vi "update unit ID.vi"(8 "error in (no error)":errorcluster, 11 "Modbus Module runtime in":refnum<class "Modbus Module runtime.lvclass">) -> (0 "error out":errorcluster, 3 "Modbus Module runtime out":refnum<class "Modbus Module runtime.lvclass">)   [LabVIEW 2015, in "Modbus Module runtime.lvclass"]
uses:
  Modbus Module runtime.lvclass
  Modbus Module runtime.lvclass/Modbus Module runtime.ctl
  <vilib>/NI/Modbus Library/API/Modbus API.lvclass/Modbus API.ctl
  <vilib>/NI/Modbus Library/Transmission Data Unit/Transmission Data Unit.lvclass/Transmission Data Unit.ctl
  <vilib>/NI/Modbus Library/Transmission Data Unit/Transmission Data Unit.lvclass
  <vilib>/NI/Modbus Library/API/Modbus API.lvclass
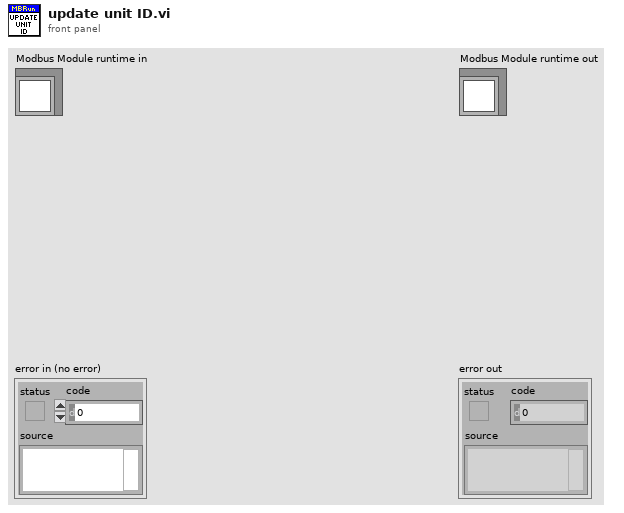
[diagram p1: front panel]
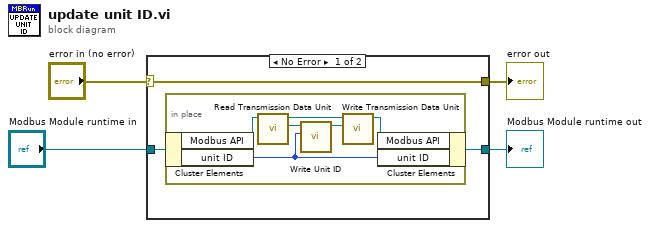
[diagram p0: block diagram]
diagram:
  n1 = case shown="No Error" "error in (no error)" {
    selector: "error in (no error)" -> [w7 w15]
    tunnel: [w7 w15] -> w3
    tunnel: [w5 w14] -> w1
    tunnel: "Modbus Module runtime in" -> [w6 w14]
    frame No Error {
      n2 = in-place {
        n3 = in-place-cluster #1(w6) -> ("Modbus API"=w13:refnum<class "Modbus API.lvclass">, "unit ID"=w8:u8)
        n4 = call <vilib>:"Read Transmission Data Unit.vi"("Modbus instance in"=w13) -> ("transmission data unit"=w12:refnum<class "Transmission Data Unit.lvclass">, "Modbus instance out"=w10:refnum<class "Modbus API.lvclass">)  [unwired: 8 in, 1 out]
        n5 = call <vilib>:"Write Unit ID.vi"("unit ID"=w8, "transmission data unit in"=w12) -> ("transmission data unit out"=w11:refnum<class "Transmission Data Unit.lvclass">)  [unwired: 8 in, 1 out]
        n6 = call <vilib>:"Write Transmission Data Unit.vi"("transmission data unit"=w11, "Modbus instance in"=w10) -> ("Modbus instance out"=w9:refnum<class "Modbus API.lvclass">)  [unwired: 8 in, 1 out]
        n7 = in-place-cluster #1("Modbus API"=w9, "unit ID"=w8) -> (w5:refnum<class "Modbus Module runtime.lvclass">)
      }
    }
    frame Error {
    }
  }
  "error out" <- w3
  "Modbus Module runtime out" <- w1
